vi "Read Data.vi"(7 "初始化?":bool, 8 "error in (no error)":errorcluster caption="错误输入（无错误）", 11 "2601B 输入":refnum<class "2601B.lvclass">) -> (0 "error out":errorcluster caption="错误输出", 1 "完成":bool, 2 "DBL":dbl[][](array[numeric]), 3 "2601B 输出":refnum<class "2601B.lvclass">)   [LabVIEW 2020, in "2601B.lvclass"]
uses:
  2601B.lvclass
  2601B.lvclass/2601B.ctl
  <vilib>/ErrorRing/Error Ring.xnode
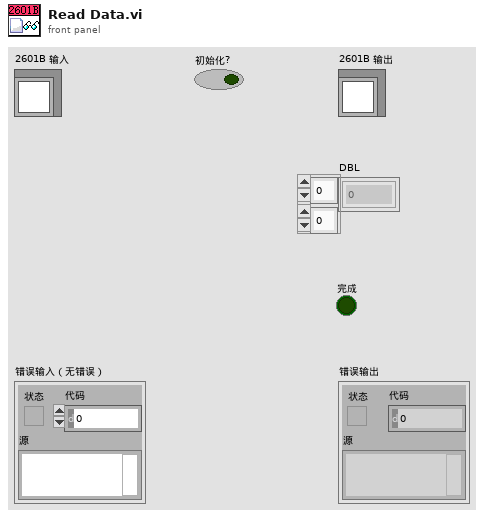
[diagram p1: front panel]
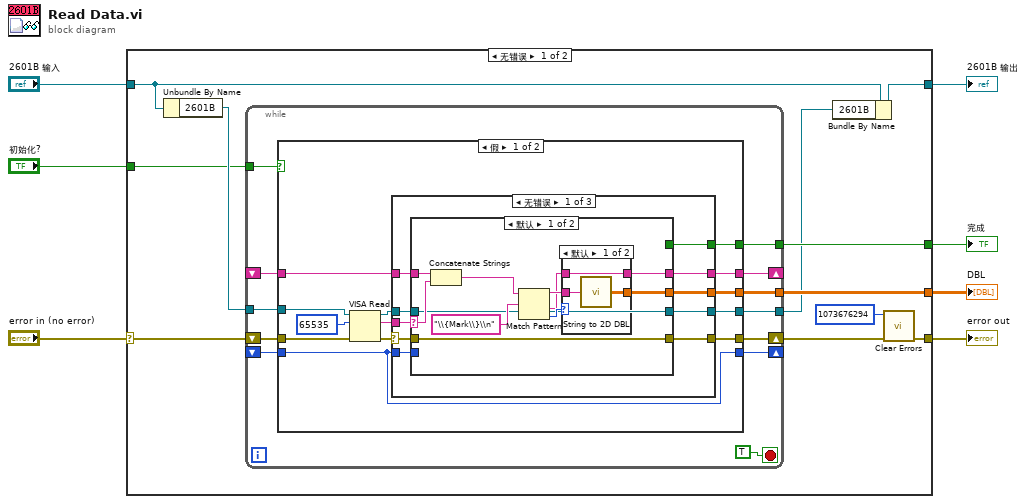
[diagram p0: block diagram]
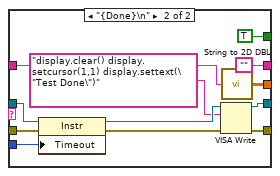
[diagram p3: hidden frame]
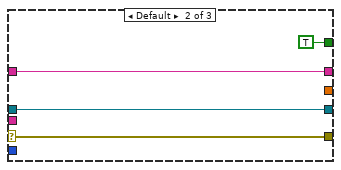
[diagram p4: hidden frame]
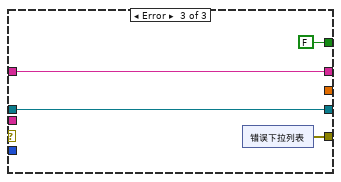
[diagram p5: hidden frame]
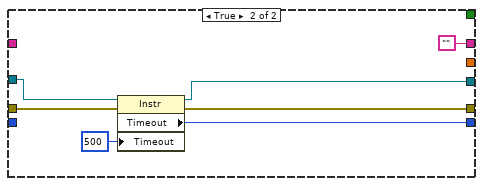
[diagram p6: hidden frame]
diagram:
  n1 = case shown="无错误" "error in (no error)" {
    selector: "error in (no error)" -> [w18 w98]
    tunnel: [w9 w98] -> w6
    tunnel: [w11 w97] -> w4
    tunnel: "2601B 输入" -> [w15 w97]
    tunnel: [w16 _] -> w3
    tunnel: [w13 _] -> w2
    tunnel: "初始化?" -> [w12 _]
    frame No Error {
      n2 = Unbundle By Name(w15) -> ("2601B"=w14:refnum<visa-resource-name>)
      n3 = while {
        shift-right: [w30] -> w17
        shift-left: w18 -> [w29]
        shift-right: [w28] -> _
        shift-left: _ -> [w22]
        tunnel: [w27] -> w16
        tunnel: w14 -> [w26]
        tunnel: [w24] -> w13
        tunnel: w12 -> [w23]
        tunnel: [w21] -> w10
        shift-right: [w20] -> _
        shift-left: _ -> [w19]
        stop <- TRUE stop-if-true
        n4 = case shown="假" w23 {
          tunnel: [w42 w94] -> w30
          tunnel: w29 -> [w41 w95]
          tunnel: [w39 ""] -> w28
          tunnel: [w38 _] -> w27
          tunnel: w26 -> [w37 w93]
          tunnel: [w36 _] -> w24
          tunnel: w22 -> [w35 _]
          tunnel: [w33 w91] -> w21
          tunnel: [w32 w90] -> w20
          tunnel: w19 -> [w32 _]
          frame False {
            n5 = VISA Read(VISA resource name=w37, byte count=u32 65535 ("字节总数"), error in (no error)=w41) -> (VISA resource name out=w34:refnum<visa-resource-name>, read buffer=w31:string, error out=w43:errorcluster)  [unwired: 1 out]
            n6 = case shown="无错误" w43 {
              selector: w43 -> [w51 w84 _]
              tunnel: [w53 TRUE FALSE] -> w36
              tunnel: [w52 w84 w87] -> w42
              tunnel: w31 -> [w50 _ _]
              tunnel: w35 -> [w49 w82 w86]
              tunnel: [w48 w82 w86] -> w39
              tunnel: [w47 _ _] -> w38
              tunnel: w34 -> [w46 w81 w85]
              tunnel: [w45 w81 w85] -> w33
              tunnel: w32 -> [w44 _ _]
              frame No Error {
                n7 = case shown="默认" w50 {
                  selector: w50 -> [w58 _]
                  tunnel: [_ TRUE] -> w53
                  tunnel: [w64 w72] -> w52
                  tunnel: w51 -> [w64 w79]
                  tunnel: w49 -> [w57 w77]
                  tunnel: [w56 ""] -> w48
                  tunnel: [w55 w76] -> w47
                  tunnel: w46 -> [w54 w74]
                  tunnel: [w54 w70] -> w45
                  tunnel: w44 -> [_ w73]
                  frame Default {
                    n8 = Concatenate Strings(w57, w58) -> (w63:string)
                    n9 = Match Pattern(string=w63, regular expression="\\{Mark\\}\\n" ("正则表达式")) -> (before substring=w60:string, after substring=w59:string, offset past match=w61:i32)  [unwired: 1 in, 1 out]
                    n10 = case shown="默认" w61 {
                      tunnel: w60 -> [w66 w68]
                      tunnel: [w65 w68] -> w56
                      tunnel: [w67 _] -> w55
                      tunnel: w59 -> [w65 _]
                      frame Default {
                        n11 = call "String to 2D DBL.vi"("String"=w66) -> ("DBL"=w67:dbl[][])
                      }
                      frame -1 {
                      }
                    }
                  }
                  frame "{Done}\n" {
                    n12 = property class="Instr"(reference=w74, error in=w79, "Timeout"=w73) -> (reference out=w71:refnum<visa-resource-name>, error out=w75:errorcluster)
                    n13 = VISA Write(VISA resource name=w71, write buffer="display.clear() display.setcursor(1,1) display.settext(\"Test Done\")", error in (no error)=w75) -> (VISA resource name out=w70:refnum<visa-resource-name>, error out=w72:errorcluster)  [unwired: 1 out]
                    n14 = call "String to 2D DBL.vi"("String"=w77) -> ("DBL"=w76:dbl[][])
                  }
                }
              }
              frame Default {
              }
              frame Error {
                n15 = xnode "错误下拉列表"() -> ("错误输出"=w87:errorcluster)
              }
            }
          }
          frame True {
            n16 = property class="Instr"(reference=w93, error in=w95, "Timeout"=u32 500 ("General Settings:Timeout Value")) -> (reference out=w91:refnum<visa-resource-name>, error out=w94:errorcluster, "Timeout"=w90:u32)
          }
        }
      }
      n17 = Bundle By Name(cluster=w15, "2601B"=w10) -> (w11:refnum<class "2601B.lvclass">)
      n18 = call <vilib>:"Clear Errors.vi"("error in (no error)"=w17, "specific error code to clear (0: all)"=1073676294) -> ("error out"=w9:errorcluster)  [unwired: 4 in, 1 out]
    }
    frame Error {
    }
  }
  "error out" <- w6
  "2601B 输出" <- w4
  "DBL" <- w3
  "完成" <- w2
